vi "Switched DAQ Wrapper.vi"(7 "Control":T2=enum."Aquire", 8 "error in":errorcluster, 10 "Config":T1={"min value"=-5.0, "max value"=5.0, "rate"=1000.0, "samples per channel"=100} {"rate" format="%#_13g"; "max value" format="%#_13g"; "min value" format="%#_13g"}, 11 "Socket":string="0") -> (0 "error out":errorcluster, 3 "AI Dataset":cluster{"Channel":string, "Data":dbl}[](array[cluster]))   [LabVIEW 2021]
uses:
  Controls/DAQ States.ctl
  Load INI/Controls/DAQ_Data.ctl
  Load INI/Controls/MUX_Data.ctl
  Controls/DataSet TypeDef.ctl
  <vilib>/numeric/Random Number (Range) DBL.vi
  <instrlib>/niSwitch/niSwitch.llb/niSwitch Connect Channels (Multiple).vi
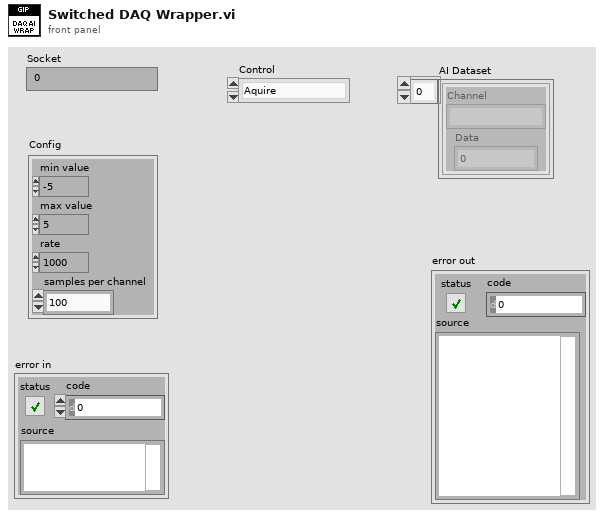
[diagram p1: front panel]
types:
  T1 = cluster{"min value":dbl, "max value":dbl, "rate":dbl, "samples per channel":i32}
  T2 = typedef "DAQ States.ctl" = enum16{"Init", "Aquire", "Close"}
  T3 = typedef "MUX_Data.ctl" = cluster{"Alias":string, "Topology":string}
  T4 = typedef "DAQ_Data.ctl" = cluster{"Alias":string, "MUX":string, "Route":string, "Channel":string}
  T5 = typedef "DataSet TypeDef.ctl" = cluster{"Channel":string, "Data":dbl}
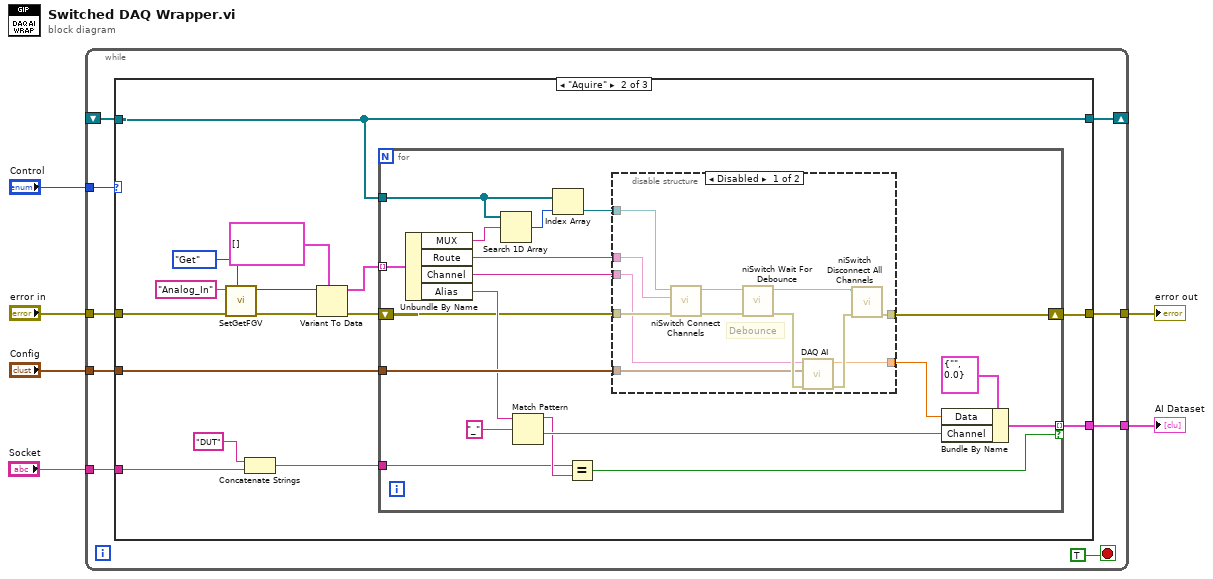
[diagram p0: block diagram]
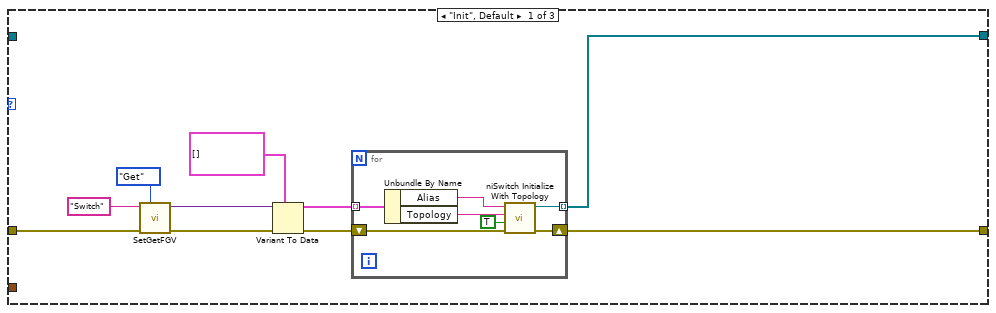
[diagram p2: hidden frame]
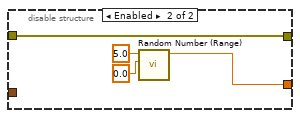
[diagram p3: hidden frame]
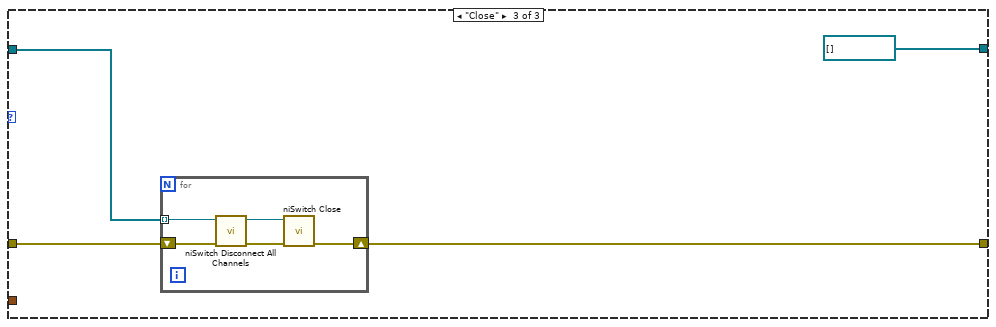
[diagram p4: hidden frame]
diagram:
  n1 = while {
    tunnel: "Control" -> [w15]
    shift-right: [w11] -> _
    shift-left: _ -> [w10]
    tunnel: "Socket" -> [w9]
    tunnel: "Config" -> [w8]
    tunnel: [w7] -> w1
    tunnel: "error in" -> [w14]
    tunnel: [w13] -> w4
    stop <- TRUE stop-if-true
    n2 = case shown="\"Aquire\"" w15 {
      tunnel: w14 -> [w25 w46 w86]
      tunnel: [w18 w47 refnum<k15>[] []] -> w11
      tunnel: w10 -> [_ w47 w84]
      tunnel: [w17 w44 w85] -> w13
      tunnel: w9 -> [_ w35 _]
      tunnel: w8 -> [_ w45 _]
      tunnel: [_ w37 _] -> w7
      frame "Init", Default {
        n3 = call "SetGetFGV.vi"("Method (Get)"=enum16{"Get", "Set"}."Get", "error in"=w25, "FGVname"="Switch") -> ("error out"=w23:errorcluster, "Data out"=w22:variant)  [unwired: 7 in]
        n4 = Variant To Data(error in=w23, type=T3[] [], Variant=w22) -> (data=w19:T3[], error out=w20:errorcluster)
        n5 = for {
          tunnel: w19 -> [w31] mode=indexing
          tunnel: [w28] -> w18 mode=indexing
          shift-right: [w27] -> w17
          shift-left: w20 -> [w32]
          n6 = Unbundle By Name(w31) -> ("Alias"=w30:string, "Topology"=w29:string)
          n7 = call <instrlib>:"niSwitch Initialize With Topology.vi"("error in (no error)"=w32, "reset device (boolean value)"=TRUE, "topology name"=w29, "resource name"=w30) -> ("error out"=w27:errorcluster, "instrument handle out"=w28:refnum<k15>)  [unwired: 6 in]
        }
      }
      frame "Aquire" {
        n8 = call "SetGetFGV.vi"("Method (Get)"=enum16{"Get", "Set"}."Get", "error in"=w46, "FGVname"="Analog_In") -> ("error out"=w41:errorcluster, "Data out"=w42:variant)  [unwired: 7 in]
        n9 = Concatenate Strings("DUT" ("string"), w35) -> (w33:string)
        n10 = Variant To Data(error in=w41, type=T4[] [], Variant=w42) -> (data=w39:T4[], error out=w38:errorcluster)
        n11 = for {
          tunnel: w39 -> [w66] mode=indexing
          tunnel: w47 -> [w53]
          tunnel: w33 -> [w58]
          tunnel: w45 -> [w61]
          shift-right: [w57] -> w44
          shift-left: w38 -> [w56]
          tunnel: [w51] -> w37 mode=indexing if=w50
          n12 = Unbundle By Name(w66) -> ("MUX"=w54:string, "Route"=w65:string, "Channel"=w64:string, "Alias"=w60:string)
          n13 = Search 1D Array(1D array=w53, element=w54) -> (index of element=w55:i32)  [unwired: 1 in]
          n14 = Match Pattern(string=w60, regular expression="_") -> (before substring=w59:string, after substring=w62:string)  [unwired: 1 in, 2 out]
          n15 = Index Array(array=w53, index=w55) -> (element=w52:refnum<k15>)
          n16 = Equal?(x=w58, y=w59) -> (x = y?=w50:bool)
          n17 = disable-structure shown="Disabled" {
            disable-tunnel: w56 -> [w77 w80]
            disable-tunnel: w65 -> [w76 _]
            disable-tunnel: w61 -> [w71 _]
            disable-tunnel: w64 -> [w70 _]
            disable-tunnel: [w69 w80] -> w57
            disable-tunnel: [w68 w79] -> w49
            disable-tunnel: w52 -> [w67 _]
            frame Disabled {
              # "Debounce"
              n18 = call-poly <instrlib>:"niSwitch Connect Channels.vi"("error in (no error)"=w77, "connection list"=w76, "instrument handle"=w67) -> ("error out"=w78:errorcluster, "instrument handle out"=w75:refnum<k15>)  [unwired: 7 in]
              n19 = call <instrlib>:"niSwitch Wait For Debounce.vi"("error in (no error)"=w78, "instrument handle"=w75) -> ("error out"=w73:errorcluster, "instrument handle out"=w74:refnum<k15>)  [unwired: 1 in, 7 out]
              n20 = call "DAQ AI.vi"("error in"=w73, "Config"=w71, "Alias"=w70) -> ("error out"=w72:errorcluster, "Data"=w68:dbl)  [unwired: 7 in]
              n21 = call <instrlib>:"niSwitch Disconnect All Channels.vi"("error in (no error)"=w72, "instrument handle"=w74) -> ("error out"=w69:errorcluster)  [unwired: 8 in, 1 out]
            }
            frame Enabled {
              n22 = call-poly <vilib>:"Random Number (Range).vi"("lower bound (0)"=0.0, "upper bound (100)"=5.0) -> ("number"=w79:dbl)  [unwired: 9 in]
            }
          }
          n23 = Bundle By Name(cluster=T5 {"Channel"="", "Data"=0.0} ("DataSet"), "Data"=w49, "Channel"=w62) -> (w51:T5)
        }
      }
      frame "Close" {
        n24 = for {
          tunnel: w84 -> [w87] mode=indexing
          shift-right: [w88] -> w85
          shift-left: w86 -> [w91]
          n25 = call <instrlib>:"niSwitch Disconnect All Channels.vi"("error in (no error)"=w91, "instrument handle"=w87) -> ("error out"=w89:errorcluster, "instrument handle out"=w90:refnum<k15>)  [unwired: 8 in]
          n26 = call <instrlib>:"niSwitch Close.vi"("error in (no error)"=w89, "instrument handle"=w90) -> ("error out"=w88:errorcluster)  [unwired: 9 in]
        }
      }
    }
  }
  "error out" <- w4
  "AI Dataset" <- w1
